vi "Add Letter.vi"(1 "String":string) -> (0 "output string":string)   [LabVIEW 2016, in "Data.lvclass"]
uses:
  Data.lvclass
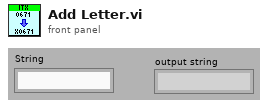
[diagram p1: front panel]
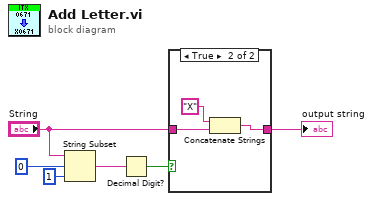
[diagram p0: block diagram]
diagram:
  n1 = String Subset(string="String", offset (0)=0, length (rest)=1 ("length (rest)")) -> (substring=w4:string)
  n2 = Decimal Digit?(1:w4) -> (0:w3:bool)
  n3 = case shown="True" w3 {
    tunnel: "String" -> [w7 w10]
    tunnel: [w7 w9] -> w1
    frame False {
    }
    frame True {
      n4 = Concatenate Strings("X", w10) -> (w9:string)
    }
  }
  "output string" <- w1
